vi "picoharp_set_sync_settings.vi"(8 "error in (no error)":errorcluster, 10 "sync_settings":T1 {"snc_offs" min=-99999 max=99999 step=1; "snc_ZeroX" min=0 max=20 step=1; "snc_level" min=0 max=800 step=10}, 11 "hydraharp in":refnum<class "picoharp.lvclass">) -> (0 "error out":errorcluster, 3 "hydraharp out":refnum<class "picoharp.lvclass">)   [LabVIEW 2015, in "picoharp.lvclass"]
uses:
  picoharp.lvclass
  Hydraharp/hydraharp_panel/hpanel_sync_settings.ctl
  Hydraharp/hydraharp_panel/hpanel_sync_div.ctl
  picoharp.lvclass/picoharp.ctl
  phlib.dll
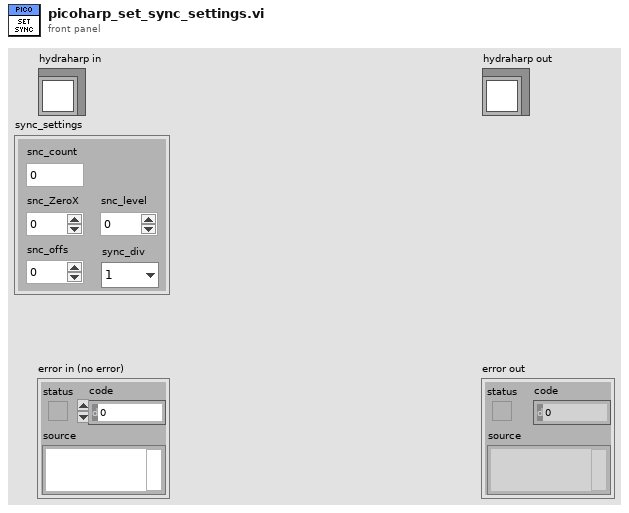
[diagram p1: front panel]
types:
  T1 = typedef "hpanel_sync_settings.ctl" = cluster{"snc_count":i32, "snc_level":i32, "snc_ZeroX":i32, "snc_offs":i32, "sync_div":T2}
  T2 = typedef "hpanel_sync_div.ctl" = enum16{"1", "2", "4", "8"}
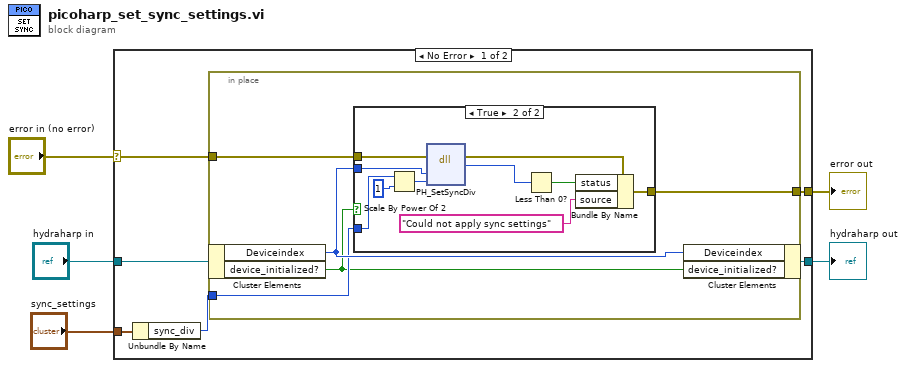
[diagram p0: block diagram]
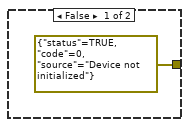
[diagram p2: hidden frame]
diagram:
  n1 = case shown="No Error" "error in (no error)" {
    selector: "error in (no error)" -> [w10 w29]
    tunnel: [w9 w29] -> w4
    tunnel: [w6 w28] -> w2
    tunnel: "hydraharp in" -> [w11 w28]
    tunnel: "sync_settings" -> [w8 _]
    frame No Error {
      n2 = Unbundle By Name(w8) -> ("sync_div"=w7:T2)
      n3 = in-place {
        in-place-border: w10 -> [w16]
        in-place-border: [w15] -> w9
        in-place-border: w7 -> [w13]
        n4 = in-place-cluster #1(w11) -> ("Deviceindex"=w14:i32, "device_initialized?"=w12:bool)
        n5 = case shown="True" w12 {
          tunnel: w16 -> [_ w19]
          tunnel: [errorcluster {"status"=TRUE, "code"=0, "source"="Device not initialized"} ("error out") w20] -> w15
          tunnel: w14 -> [_ w26]
          tunnel: w13 -> [_ w24]
          frame False {
          }
          frame True {
            n6 = Scale By Power Of 2(n=w24, x=1) -> (x*2^n=w23:i32)
            n7 = dll-call lib="phlib.dll" fn="PH_SetSyncDiv" label="pH_SetSyncDiv"(error in=w19, "devidx"=w26, "divider"=w23) -> (error out=w22:errorcluster, "return type"=w27:i32)  [unwired: 4 in, 1 out]
            n8 = Less Than 0?(x=w27) -> (x < 0?=w18:bool)
            n9 = Bundle By Name(cluster=w22, "status"=w18, "source"="Could not apply sync settings") -> (w20:errorcluster)
          }
        }
        n10 = in-place-cluster #1("Deviceindex"=w14, "device_initialized?"=w12) -> (w6:refnum<class "picoharp.lvclass">)
      }
    }
    frame Error {
    }
  }
  "error out" <- w4
  "hydraharp out" <- w2
